vi "OpenShortCompensation.vi"(9 "additional frequencies":dbl[](array[numeric]) format="%#_6p", 10 "resource name":refnum<k15>, 11 "file path (dialog if empty)":path) -> (0 "error out":errorcluster, 3 "compensation data":u8[](array[numeric]))   [LabVIEW 2023]
uses:
  <vilib>/Utility/file.llb/Write Delimited Spreadsheet (I64).vi
panel:
  in  "Start":bool
  in  "stop":bool
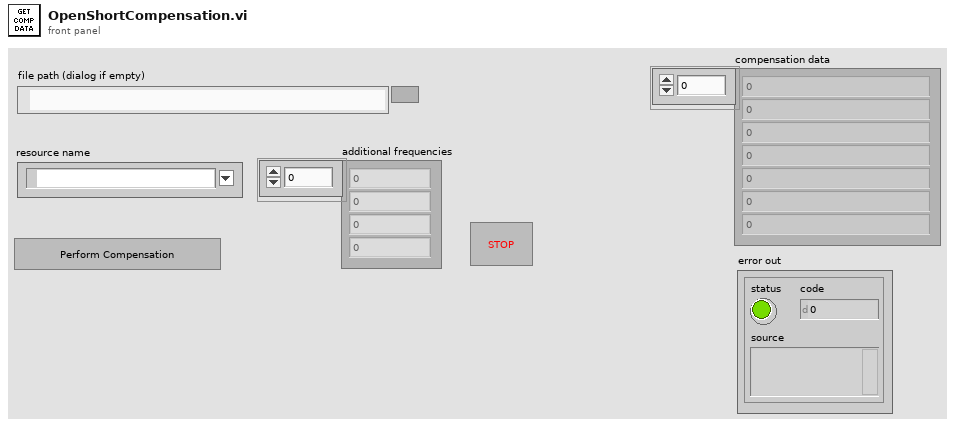
[diagram p1: front panel]
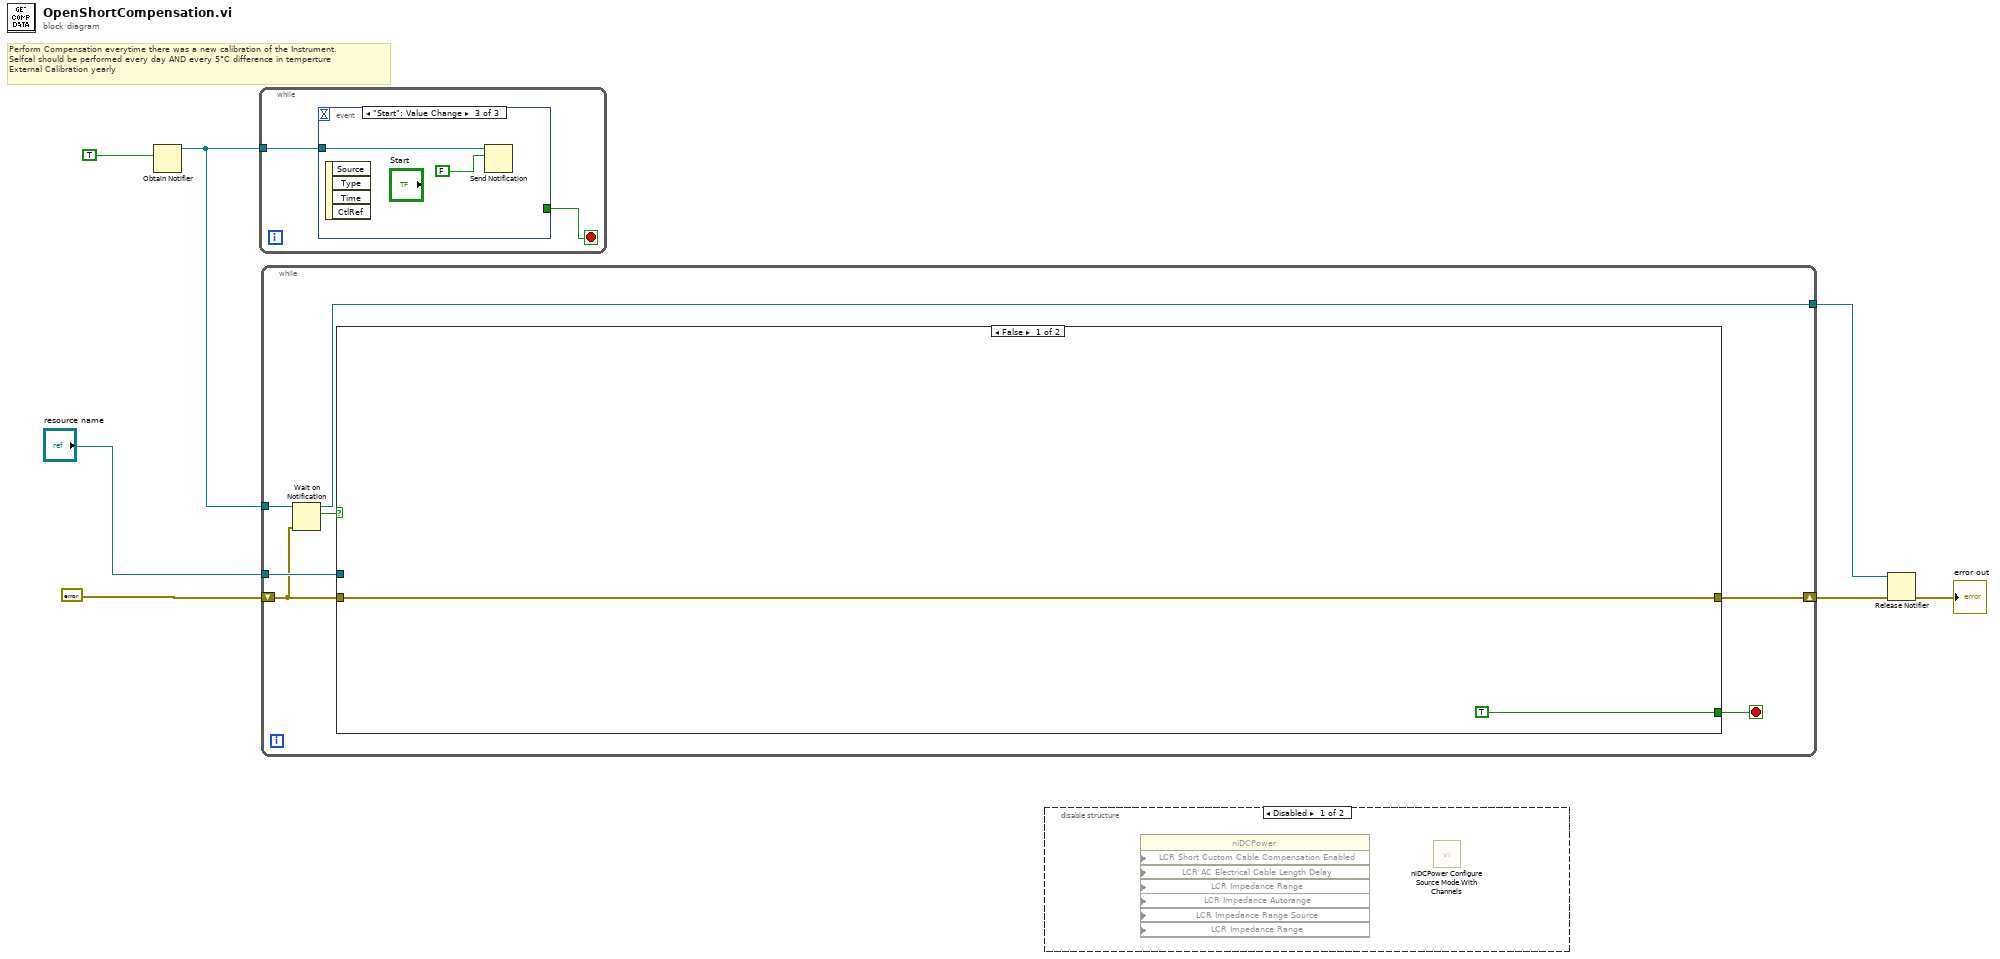
[diagram p0: block diagram]
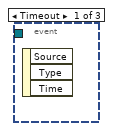
[diagram p2: hidden frame]
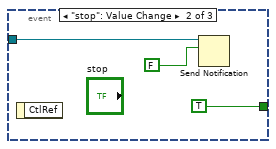
[diagram p3: hidden frame]
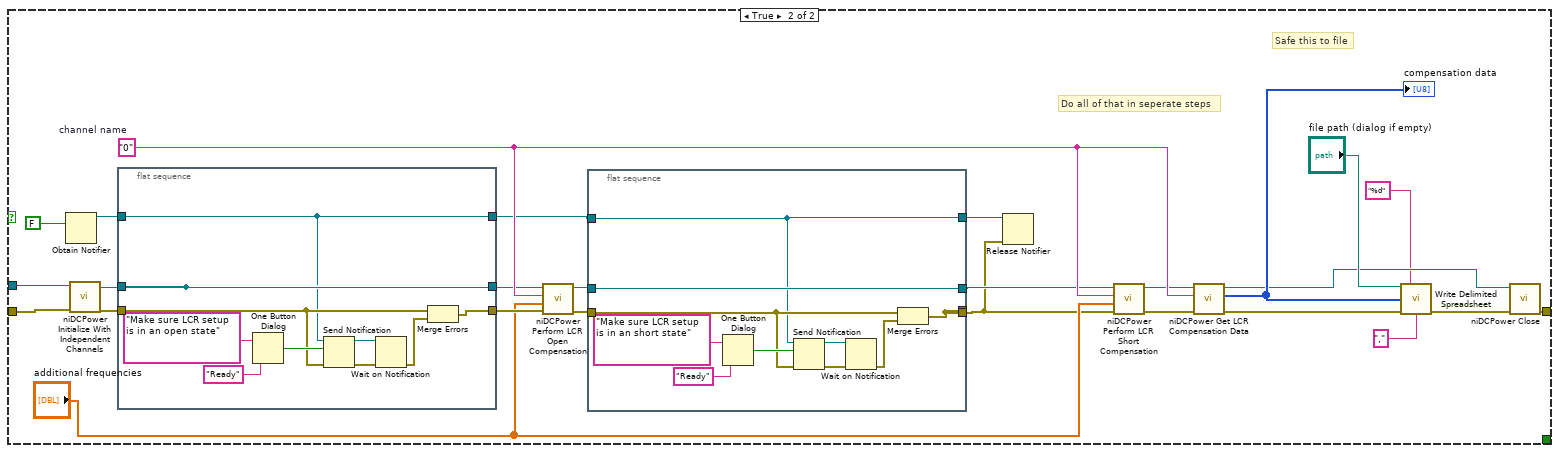
[diagram p4: hidden frame]
diagram:
  # "Perform Compensation everytime there was a new calibration of the Instrument.\nSelfcal should be performed every day AND every 5°C difference in temperture\nExternal Calibration yearly"
  n1 = Obtain Notifier(notification data type=TRUE) -> (notifier out=w4:refnum<notifier>)  [unwired: 3 in, 2 out]
  n2 = while {
    tunnel: w4 -> [w8]
    stop <- w9 stop-if-true
    n3 = event shown="[2] \"Start\": Value Change" {
      selector: _ -> [_ _ _]
      dyn-events: _ -> [_ _ _]
      timeout: _ -> [_ _ _]
      tunnel: [_ TRUE _] -> w9
      tunnel: w8 -> [_ w10 w13]
      event Timeout {
        n4 = event-data() -> ()  [unwired: 1 in, 3 out]
      }
      event "stop": Value Change {
        n5 = event-data() -> ()  [unwired: 1 in, 1 out]
        n6 = Send Notification(notification=FALSE, notifier=w10) -> ()  [unwired: 1 in, 2 out]
      }
      event "Start": Value Change {
        n7 = event-data() -> ()  [unwired: 1 in, 4 out]
        n8 = Send Notification(notification=FALSE, notifier=w13) -> ()  [unwired: 1 in, 2 out]
      }
    }
  }
  n9 = while {
    tunnel: "resource name" -> [w21]
    shift-right: [w20] -> w2
    shift-left: errorcluster {"status"=FALSE, "code"=0, "source"=""} ("error in (no error)") -> [w17]
    tunnel: w4 -> [w18]
    tunnel: [w15] -> w3
    stop <- w19 stop-if-true
    n10 = Wait on Notification(notifier=w18, error in (no error)=w17) -> (notifier out=w15:refnum<notifier>, notification=w16:bool)  [unwired: 2 in, 2 out]
    n11 = case shown="False" w16 {
      tunnel: w21 -> [_ w48]
      tunnel: w17 -> [w22 w47]
      tunnel: [w22 w27] -> w20
      tunnel: [TRUE _] -> w19
      frame False {
      }
      frame True {
        w46 = "0"  # channel name
        # "Safe this to file"
        # "Do all of that in seperate steps"
        n12 = Obtain Notifier(notification data type=FALSE ("true")) -> (notifier out=w33:refnum<notifier>)  [unwired: 3 in, 2 out]
        n13 = call <instrlib>:"niDCPower Initialize With Independent Channels.vi"("error in (no error)"=w47, "resource name"=w48) -> ("error out"=w35:errorcluster, "instrument handle out"=w36:refnum<k15>)  [unwired: 8 in]
        n14 = flat-sequence {
          tunnel: w36 -> [w68]
          tunnel: [w60] -> w34
          tunnel: w35 -> [w61]
          tunnel: [w68] -> _
          tunnel: w33 -> [w59]
          tunnel: [w59] -> w31
          frame #0 {
            n15 = One Button Dialog(message="Make sure LCR setup is in an open state", button name ("OK")="Ready") -> (true=w65:bool)
            n16 = Send Notification(notification=w65, notifier=w59, error in (no error)=w61) -> (notifier out=w64:refnum<notifier>, error out=w63:errorcluster)
            n17 = Wait on Notification(notifier=w64, error in (no error)=w63) -> (error out=w62:errorcluster)  [unwired: 2 in, 3 out]
            n18 = Merge Errors(w61, w62) -> (w60:errorcluster)
          }
        }
        n19 = call <instrlib>:"niDCPower Perform LCR Open Compensation.vi"("error in (no error)"=w34, "additional frequencies"="additional frequencies", "channel name"=w46, "instrument handle"=w36) -> ("error out"=w29:errorcluster, "instrument handle out"=w30:refnum<k15>)  [unwired: 6 in]
        n20 = flat-sequence {
          tunnel: w30 -> [w58]
          tunnel: [w50] -> _
          tunnel: w29 -> [w51]
          tunnel: [w58] -> w28
          tunnel: w31 -> [w49]
          tunnel: [w50] -> w25
          tunnel: [w49] -> w24
          frame #0 {
            n21 = One Button Dialog(message="Make sure LCR setup is in an short state", button name ("OK")="Ready") -> (true=w55:bool)
            n22 = Send Notification(notification=w55, notifier=w49, error in (no error)=w51) -> (notifier out=w54:refnum<notifier>, error out=w53:errorcluster)
            n23 = Wait on Notification(notifier=w54, error in (no error)=w53) -> (error out=w52:errorcluster)  [unwired: 2 in, 3 out]
            n24 = Merge Errors(w51, w52) -> (w50:errorcluster)
          }
        }
        n25 = Release Notifier(notifier=w24, error in (no error)=w25) -> ()  [unwired: 1 in, 3 out]
        n26 = call <instrlib>:"niDCPower Perform LCR Short Compensation.vi"("error in (no error)"=w25, "additional frequencies"="additional frequencies", "channel name"=w46, "instrument handle"=w28) -> ("error out"=w45:errorcluster, "instrument handle out"=w44:refnum<k15>)  [unwired: 6 in]
        n27 = call <instrlib>:"niDCPower Get LCR Compensation Data.vi"("error in (no error)"=w45, "channel name"=w46, "instrument handle"=w44) -> ("error out"=w40:errorcluster, "compensation data"=w41:u8[], "instrument handle out"=w38:refnum<k15>)  [unwired: 6 in]
        "compensation data" <- w41
        n28 = call-poly <vilib>:"Write Delimited Spreadsheet.vi"("file path (dialog if empty)"="file path (dialog if empty)", "format (%d)"="%d", "1D data"=w41, "error in (no error)"=w40, "delimiter (\\t)"="," ("delimiter (\\t)")) -> ("error out"=w39:errorcluster)  [unwired: 9 in, 1 out]
        n29 = call <instrlib>:"niDCPower Close.vi"("error in (no error)"=w39, "instrument handle"=w38) -> ("error out"=w27:errorcluster)  [unwired: 9 in]
      }
    }
  }
  n30 = disable-structure shown="Disabled" {
    frame Disabled {
      n31 = property class="niDCPower" props=["LCR Short Custom Cable Compensation Enabled", "LCR AC Electrical Cable Length Delay", "LCR Impedance Range", "LCR Impedance Autorange", "LCR Impedance Range Source", "LCR Impedance Range"]() -> ()  [unwired: 8 in, 2 out]
      n32 = call <instrlib>:"niDCPower Configure Source Mode With Channels.vi"() -> ()  [unwired: 10 in, 2 out]
    }
    frame Enabled {
    }
  }
  n33 = Release Notifier(notifier=w3, error in (no error)=w2) -> (error out=→"error out":errorcluster)  [unwired: 1 in, 2 out]
